vi "setPathAndType.vi"(8 "error in (no error)":errorcluster, 9 "fileType":T1, 10 "Path":path, 11 "reference in":refnum<class "excelFile.lvclass">) -> (0 "error out":errorcluster, 3 "reference out":refnum<class "excelFile.lvclass">)   [LabVIEW 2015, in "excelFile.lvclass"]
uses:
  excelFile.lvclass
  fileType.ctl
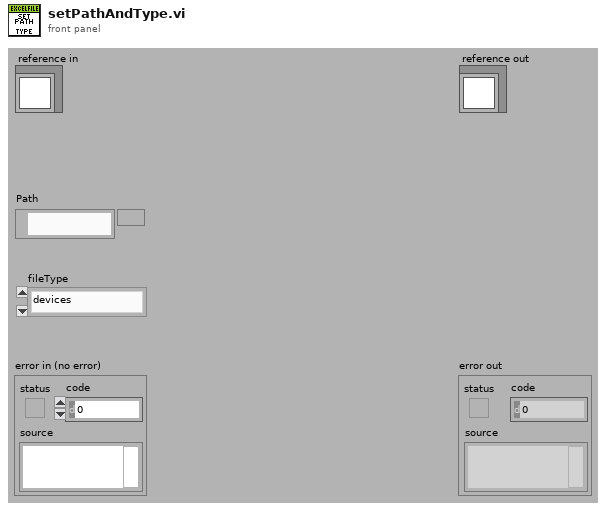
[diagram p1: front panel]
types:
  T1 = typedef "excelFile.lvclass/fileType.ctl" = enum16{"devices", "items", "partsTracking", "TSR"}
  T2 = typedef "excelFile.lvclass/ObjectAttributesRef.ctl" = refnum<data-value>
  T3 = typedef "excelFile.lvclass/ObjectAttributes.ctl" = cluster{"MyAttribute":dbl, "path":string, "Refnum Excel":cluster{"Excel._Application":refnum<k7>, "Workbooks":refnum<k7>, "Open":refnum<k7>}, "data":string[][][], "save":bool, "fileType":T1, "rowsColor":u32[], "python_ref":refnum<class "python.lvclass">, "items_rows":i32[], "excel_range":i32[][]}
  T4 = typedef "excelFile.lvclass/ClassAttributesRef.ctl" = refnum<data-value>
  T5 = typedef "excelFile.lvclass/ClassAttributes.ctl" = cluster{"Dummy":bool, "excelFile_refs":refnum<class "excelFile.lvclass">[]}
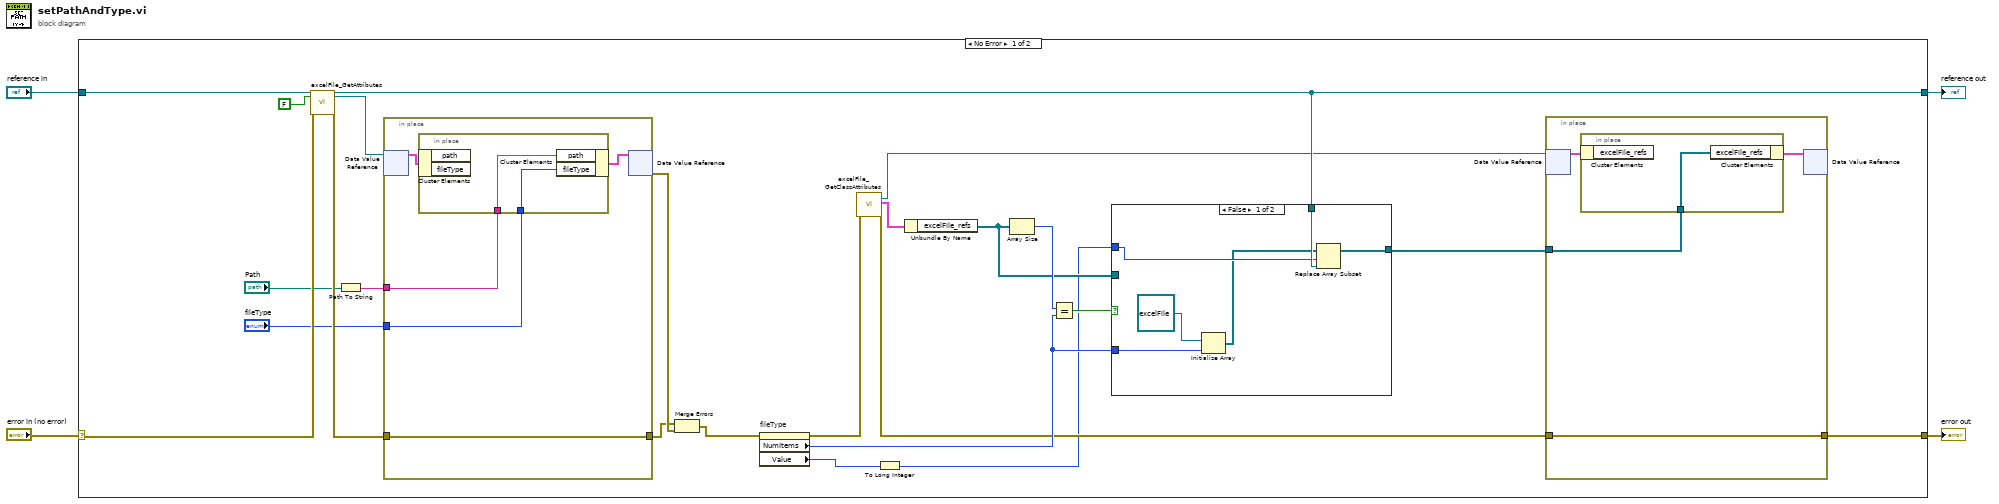
[diagram p0: block diagram]
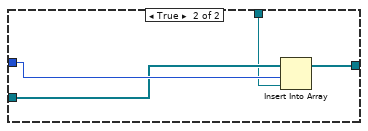
[diagram p2: hidden frame]
diagram:
  n1 = case shown="No Error" "error in (no error)" {
    selector: "error in (no error)" -> [w24 w52]
    tunnel: [w9 w52] -> w3
    tunnel: [w12 w51] -> w1
    tunnel: "reference in" -> [w26 w51]
    frame No Error {
      n2 = call "excelFile_GetAttributes.vi"("reference in"=w26, "return data? (T)"=FALSE, "error in (no error)"=w24) -> ("reference out"=w12:refnum<class "excelFile.lvclass">, "attributes ref"=w22:T2, "error out"=w23:errorcluster)  [unwired: 13 in, 1 out]
      n3 = Path To String(path="Path") -> (string=w20:string)
      n4 = in-place {
        in-place-border: w23 -> [w46]
        in-place-border: [w46] -> w27
        in-place-border: w20 -> [w45]
        in-place-border: "fileType" -> [w44]
        n5 = in-place-dvr #1(w22) -> (w47:T3)  [unwired: 1 out]
        n6 = in-place {
          in-place-border: w45 -> [w50]
          in-place-border: w44 -> [w49]
          n7 = in-place-cluster #2(w47) -> ()  [unwired: 2 out]
          n8 = in-place-cluster #2("path"=w50, "fileType"=w49) -> (w48:T3)
        }
        n9 = in-place-dvr #1(w48) -> (w28:errorcluster)  [unwired: 1 out]
      }
      n10 = Merge Errors(w27, w28) -> (w19:errorcluster)
      n11 = property on="fileType" class="Enum (strict)"(error in=w19) -> (error out=w18:errorcluster, "NumItems"=w13:u32, "Value"=w6:T1)  [unwired: 1 in, 1 out]
      n12 = call "excelFile_GetClassAttributes.vi"("error in (no error)"=w18) -> ("class attributes ref"=w8:T4, "class attributes"=w17:T5, "error out"=w10:errorcluster)  [unwired: 15 in, 1 out]
      n13 = To Long Integer(number=w6) -> (32bit integer=w5:i32)
      n14 = Unbundle By Name(w17) -> ("excelFile_refs"=w11:refnum<class "excelFile.lvclass">[])
      n15 = Array Size(array=w11) -> (size(s)=w16:i32)
      n16 = Equal?(x=w16, y=w13) -> (x = y?=w15:bool)
      n17 = case shown="False" w15 {
        tunnel: w5 -> [w36 w43]
        tunnel: w13 -> [w38 _]
        tunnel: w12 -> [w37 w41]
        tunnel: w11 -> [_ w42]
        tunnel: [w34 w40] -> w7
        frame False {
          n18 = Initialize Array(refnum<class "excelFile.lvclass"> refnum ("excelFile.lvclass"), w38) -> (w35:refnum<class "excelFile.lvclass">[])
          n19 = Replace Array Subset(array=w35, new element=w37, index=w36) -> (w34:refnum<class "excelFile.lvclass">[])
        }
        frame True {
          n20 = Insert Into Array(array=w42, index=w43, new element=w41) -> (w40:refnum<class "excelFile.lvclass">[])
        }
      }
      n21 = in-place {
        in-place-border: w10 -> [w30]
        in-place-border: [w30] -> w9
        in-place-border: w7 -> [w29]
        n22 = in-place-dvr #3(w8) -> (w31:T5)  [unwired: 1 out]
        n23 = in-place {
          in-place-border: w29 -> [w33]
          n24 = in-place-cluster #4(w31) -> ()  [unwired: 1 out]
          n25 = in-place-cluster #4("excelFile_refs"=w33) -> (w32:T5)
        }
        n26 = in-place-dvr #3(w32) -> ()  [unwired: 2 out]
      }
    }
    frame Error {
    }
  }
  "error out" <- w3
  "reference out" <- w1
